vi "WriteThrustOpenLoop.vi"(9 "Left":u16, 10 "Right":u16, 11 "Refnum in":refnum<k20>) -> (1 "PacketOut":u8[](array[numeric]))   [LabVIEW 2011]
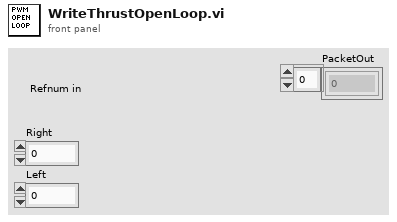
[diagram p1: front panel]
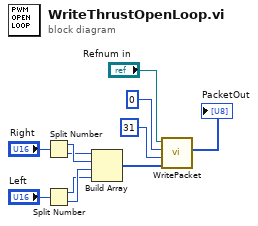
[diagram p0: block diagram]
diagram:
  n1 = Split Number(x="Right") -> (hi(x)=w8:u8, lo(x)=w7:u8)
  n2 = Split Number(x="Left") -> (hi(x)=w5:u8, lo(x)=w6:u8)
  n3 = Build Array(w7, w8, w6, w5) -> (w4:u8[])
  n4 = call "WritePacket.vi"("Payload"=w4, "Type"=u8 31, "Status"=u8 0, "Refnum in"="Refnum in") -> ("PacketOut"=→"PacketOut":u8[])  [unwired: 7 in]
